vi "NF87XX.start motion.vi"(0 "i ref in":refnum<vi>, 2 "System":string="N/A", 5 "error in (no error)":errorcluster) -> (14 "i ref out":refnum<vi>, 19 "error out":errorcluster)   [LabVIEW 2014, in "NF87XX.lvlib"]
doc: "Starts the movement with the current configuration.\n\nauthor: Stefan Götte\ndata: 09-JAN-2007\n\nLicense Agreement for this software:\n\nCopyright (C)\nGesellschaft für Schwerionenforschung, GSI\nPlanckstr. 1\n64291 Darmstadt\nGermany\n\nContact: D.Beck@gsi.de \n\nThis program is free software; you can redistribute it and/or modify it under the terms of the GNU General Public License as published by the Free Software Foundation; either version 2 of the license, or (at your option) any later version.\n\nThis program is distributed in the hope that it will be useful, but WITHOUT ANY WARRANTY; without even the implied warranty of MERCHANTABILITY or FITNESS FOR A PARTICULAR PURPOSE. See the GNU General License for more details (http://www.gnu.org).\n\nGesellschaft für Schwerionenforschung, GSI\nPlanckstr. 1, 64291 Darmstadt, Germany\nFor all questions and ideas contact: M.Richter@gsi.de, H.Brand@gsi.de or D.Beck@gsi.de.\nLast update: 17-JUN-2004"
uses:
  NF87XX.lvlib
  instr.lib/NewFocusPico/Pico Parameters.ctl
  instr.lib/NewFocusPico/NewFocusPico - Driver np.lvlib
panel:
  in  "Pico Parameter type":T1={"Pico Type"=enum."Open-Loop Pico", "Acceleration (steps/sec^2)"="32000", "Velocity ( Hz)"="2000", "Driver"="A1", "Motor"="0", "Channel"="0", "Process Step"="Final Test"}
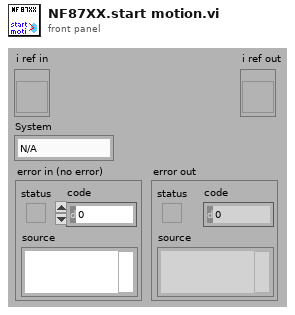
[diagram p1: front panel]
types:
  T1 = typedef "NewFocusPico - Driver np.lvlib/Pico Parameters.ctl" = cluster{"Pico Type":enum16{"Open-Loop Pico", "Close-Loop Pico", "Pico Ultra"}, "Acceleration (steps/sec^2)":string, "Velocity ( Hz)":string, "Driver":string, "Motor":string, "Channel":string, "Process Step":string}
  T2 = enum16{"User....", "DEF", "DIAG", "INI", "LOCK", "UNLOCK", "MAP", "SAV", "VER", "ACC", "CHL", "FOR", "GO", "HAL", "MOF", "MON", "MPV", "POS", "REL", "REV", "STA", "STO", "TYP", "VEL", "ABS", "SER", "NOS", "DRT", "FLI", "RLI", "FIN", "RIN", "AIN", "IN", "JOF", "JON", "OUT", "RES FINE", "RES COARSE", "02 (HEX)", "PWM", "CNT", "TMR", "HOSTNAME", "IPADDR", "IPMODE", "NETMASK", "GATEWAY", "DNSSRVR", "PASSWD", "ECHO", "MACADDR"}
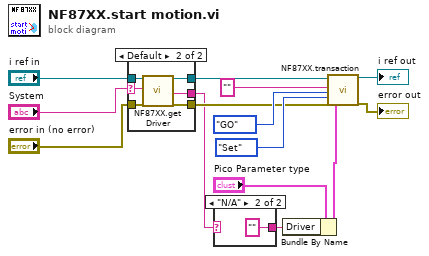
[diagram p0: block diagram]
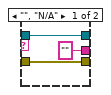
[diagram p2: hidden frame]
diagram:
  n1 = case shown="Default" "System" {
    selector: "System" -> [_ w18]
    tunnel: "i ref in" -> [w17 w23]
    tunnel: "error in (no error)" -> [w16 w22]
    tunnel: [w17 w21] -> w10
    tunnel: [w16 w20] -> w5
    tunnel: ["" ("Driver") w19] -> w1
    frame "", "N/A" {
    }
    frame Default {
      n2 = call "NF87XX.get Driver.vi"("i ref in"=w23, "System"=w18, "error in (no error)"=w22) -> ("i ref out"=w21:refnum<vi>, "Driver"=w19:string, "error out"=w20:errorcluster)  [unwired: 12 in, 2 out]
    }
  }
  n3 = case shown="\"N/A\"" w1 {
    selector: w1 -> [w24 _]
    tunnel: [w24 ""] -> w2
    frame Default {
    }
    frame "N/A" {
    }
  }
  n4 = Bundle By Name(cluster="Pico Parameter type", "Driver"=w2) -> (w6:T1)
  n5 = call "NF87XX.transaction.vi"("i ref in"=w10, "User Cmd/Numeric Argu"="", "MCL Cmd"=T2."GO", "Query/Set"=enum16{"Query", "Set"}."Set", "error in (no error)"=w5, "Pico Parameter"=w6) -> ("i ref out"=→"i ref out":refnum<vi>, "error out"=→"error out":errorcluster)  [unwired: 11 in, 1 out]
